vi "Create Side View Cavity Spark Scene.vi"(2 "error in (no error)":errorcluster, 3 "Spark Coordinates":T1) -> (0 "error out":errorcluster, 1 "reference out":refnum<vi>)   [LabVIEW 2013]
uses:
  <vilib>/Utility/miscctls.llb/LV3DPointTypeDef.ctl
  <vilib>/picture/3D Picture Control/Object/Create Object (name).vi
  <vilib>/picture/3D Picture Control/NI_3D Picture Control.lvlib
panel:
  out "Cavity Side View":refnum<vi>(3d-picture)
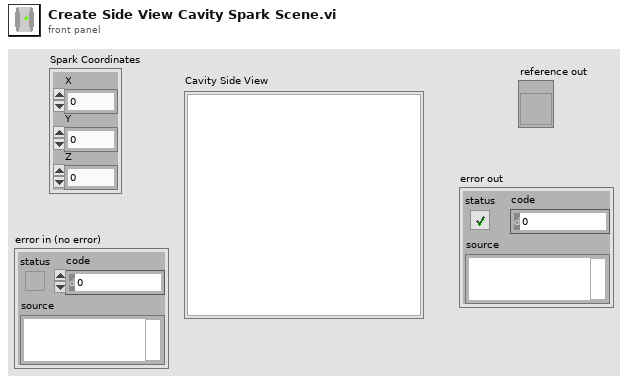
[diagram p1: front panel]
types:
  T1 = typedef "LV3DPointTypeDef.ctl" = cluster{"X":sgl, "Y":sgl, "Z":sgl}
  T2 = cluster{"Red":sgl, "Green":sgl, "Blue":sgl, "Alpha":sgl}
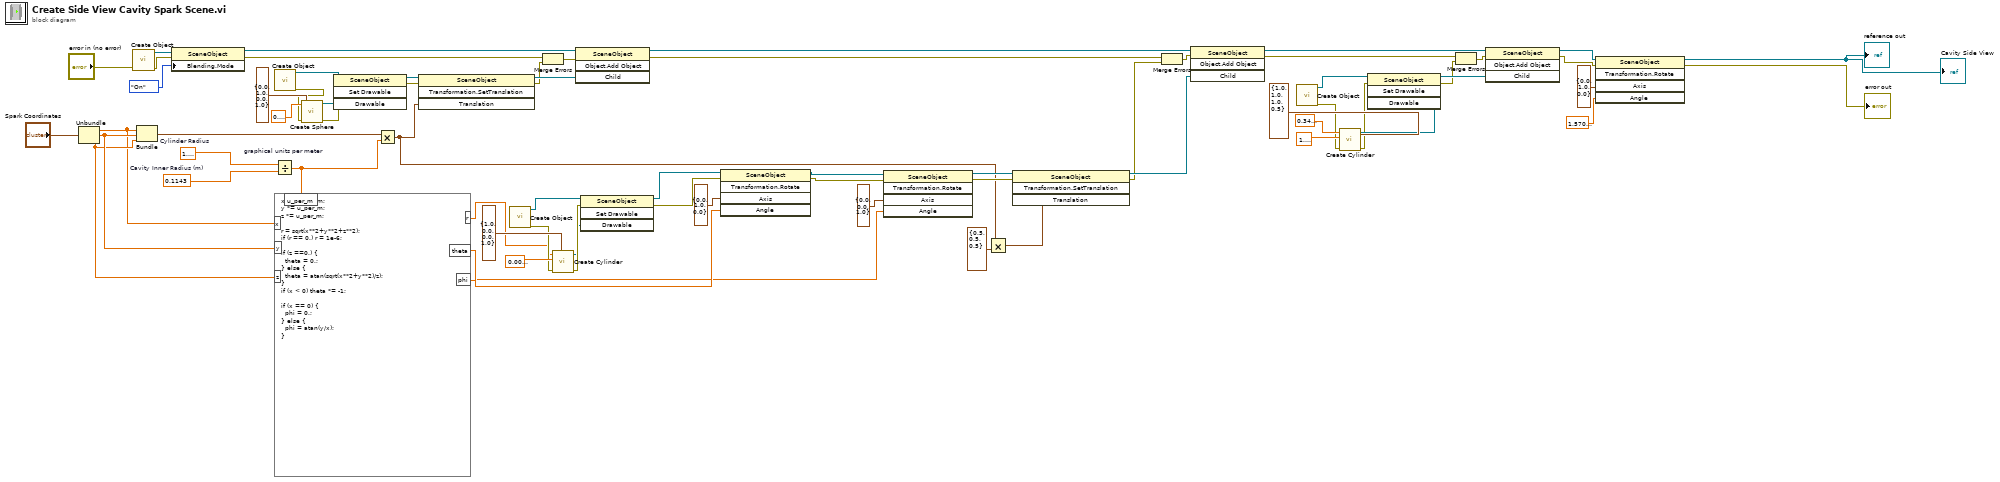
[diagram p0: block diagram]
diagram:
  w37 = 0.1143  # Cavity Inner Radius (m)
  w36 = sgl 1.2  # Cylinder Radius
  n1 = Unbundle("Spark Coordinates") -> ("X"=w4:sgl, "Y"=w28:sgl, "Z"=w27:sgl)
  n2 = call-poly <vilib>:"Create Object.vi"("error in (no error)"="error in (no error)") -> ("error out"=w65:errorcluster, "Scene:New Object"=w66:refnum<vi>)  [unwired: 9 in]
  n3 = Bundle("X"=w4, "Y"=w28, "Z"=w27) -> (w34:cluster{"X":sgl, "Y":sgl, "Z":sgl})  [unwired: 1 in]
  n4 = property class="SceneObject"(reference=w66, error in=w65, "Blending.Mode"=enum16{"Inherit Value", "Off", "On"}."On" ("Blending:Mode")) -> (reference out=w64:refnum<vi>, error out=w40:errorcluster)
  n5 = Divide "graphical units per meter"(x=w36, y=w37) -> (x/y=w18:dbl)
  n6 = call-poly <vilib>:"Create Object.vi"() -> ("error out"=w45:errorcluster, "Scene:New Object"=w53:refnum<vi>)  [unwired: 10 in]
  n7 = formula code="x *= u_per_m;\ny *= u_per_m;\nz *= u_per_m;\n\nr = sqrt(x**2+y**2+z**2);\nif (r == 0.) r = 1e-6;\n\nif (z ==0.) {\n  theta = 0.;\n} else {\n  theta = atan(sqrt(x**2+y**2)/z);\n}\nif (x < 0) theta *= -1;\n\nif (x == 0) {\n  phi = 0.;\n} else {\n  phi = atan(y/x);\n}"("x"=w4, "y"=w28, "z"=w27, "u_per_m"=w18) -> ("r"=w17:dbl, "theta"=w8:dbl, "phi"=w7:dbl)
  n8 = call <vilib>:"Create Sphere.vi"("Color"=T2 {"Red"=0.0, "Green"=1.0, "Blue"=0.0, "Alpha"=1.0}, "error in (no error)"=w45, "Radius"=sgl 0.1) -> ("error out"=w44:errorcluster, "New Sphere Refnum"=w54:refnum<vi>)  [unwired: 7 in]
  n9 = invoke class="SceneObject" method="Set Drawable"(reference=w53, error in=w44, "Drawable"=w54) -> (reference out=w52:refnum<vi>, error out=w51:errorcluster)  [unwired: 1 in, 2 out]
  n10 = Multiply(x=w34, y=w18) -> (x*y=w6:cluster{"X":dbl, "Y":dbl, "Z":dbl})
  n11 = invoke class="SceneObject" method="Transformation.SetTranslation"(reference=w52, error in=w51, "Translation"=w6) -> (reference out=w50:refnum<vi>, error out=w42:errorcluster)  [unwired: 1 in, 2 out]
  n12 = call-poly <vilib>:"Create Object.vi"() -> ("error out"=w30:errorcluster, "Scene:New Object"=w32:refnum<vi>)  [unwired: 10 in]
  n13 = Merge Errors(w40, w42) -> (w41:errorcluster)
  n14 = call <vilib>:"Create Cylinder.vi"("Color"=T2 {"Red"=1.0, "Green"=0.0, "Blue"=0.0, "Alpha"=1.0}, "error in (no error)"=w30, "Radius"=sgl 0.01, "Height"=w17) -> ("error out"=w29:errorcluster, "New Cylinder Refnum"=w19:refnum<vi>)  [unwired: 6 in]
  n15 = invoke class="SceneObject" method="Object.Add Object"(reference=w64, error in=w41, "Child"=w50) -> (reference out=w11:refnum<vi>, error out=w12:errorcluster)  [unwired: 1 in, 2 out]
  n16 = invoke class="SceneObject" method="Set Drawable"(reference=w32, error in=w29, "Drawable"=w19) -> (reference out=w15:refnum<vi>, error out=w14:errorcluster)  [unwired: 1 in, 2 out]
  n17 = invoke class="SceneObject" method="Transformation.Rotate"(reference=w15, error in=w14, "Axis"=T1 {"X"=0.0, "Y"=1.0, "Z"=0.0}, "Angle"=w8) -> (reference out=w23:refnum<vi>, error out=w22:errorcluster)  [unwired: 1 in, 3 out]
  n18 = invoke class="SceneObject" method="Transformation.Rotate"(reference=w23, error in=w22, "Axis"=T1 {"X"=0.0, "Y"=0.0, "Z"=1.0}, "Angle"=w7) -> (reference out=w21:refnum<vi>, error out=w20:errorcluster)  [unwired: 1 in, 3 out]
  n19 = Multiply(x=w6, y=cluster{"X":dbl, "Y":dbl, "Z":dbl} {"X"=0.5, "Y"=0.5, "Z"=0.5}) -> (x*y=w5:cluster{"X":dbl, "Y":dbl, "Z":dbl})
  n20 = invoke class="SceneObject" method="Transformation.SetTranslation"(reference=w21, error in=w20, "Translation"=w5) -> (reference out=w16:refnum<vi>, error out=w13:errorcluster)  [unwired: 1 in, 2 out]
  n21 = Merge Errors(w12, w13) -> (w26:errorcluster)
  n22 = invoke class="SceneObject" method="Object.Add Object"(reference=w11, error in=w26, "Child"=w16) -> (reference out=w10:refnum<vi>, error out=w9:errorcluster)  [unwired: 1 in, 2 out]
  n23 = call-poly <vilib>:"Create Object.vi"() -> ("error out"=w49:errorcluster, "Scene:New Object"=w62:refnum<vi>)  [unwired: 10 in]
  n24 = call <vilib>:"Create Cylinder.vi"("Color"=T2 {"Red"=1.0, "Green"=1.0, "Blue"=1.0, "Alpha"=0.5}, "error in (no error)"=w49, "Radius"=sgl 1.2, "Height"=sgl 0.34) -> ("error out"=w48:errorcluster, "New Cylinder Refnum"=w67:refnum<vi>)  [unwired: 6 in]
  n25 = invoke class="SceneObject" method="Set Drawable"(reference=w62, error in=w48, "Drawable"=w67) -> (reference out=w58:refnum<vi>, error out=w38:errorcluster)  [unwired: 1 in, 2 out]
  n26 = Merge Errors(w9, w38) -> (w39:errorcluster)
  n27 = invoke class="SceneObject" method="Object.Add Object"(reference=w10, error in=w39, "Child"=w58) -> (reference out=w57:refnum<vi>, error out=w47:errorcluster)  [unwired: 1 in, 2 out]
  n28 = invoke class="SceneObject" method="Transformation.Rotate"(reference=w57, error in=w47, "Axis"=T1 {"X"=0.0, "Y"=1.0, "Z"=0.0}, "Angle"=sgl 1.571) -> (reference out=→"reference out" →"Cavity Side View":refnum<vi>, error out=→"error out":errorcluster)  [unwired: 1 in, 3 out]
